vi "GetType.vi"(8 "error in (no error)":errorcluster, 11 "Set Output Voltages Msg":refnum<class "Set Output Voltages Msg.lvclass">) -> (0 "error out":errorcluster, 2 "Data Sample":variant, 3 "Set Output Voltages Msg":refnum<class "Set Output Voltages Msg.lvclass">)   [LabVIEW 2015, in "BNT_DAQmx.lvlib" / "Set Output Voltages Msg.lvclass"]
uses:
  Set Output Voltages Msg.lvclass
  Set Output Voltages Msg.lvclass/Set Output Voltages Msg.ctl
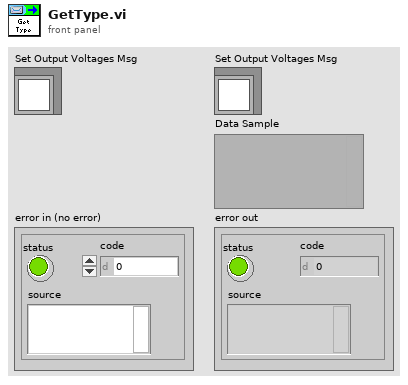
[diagram p1: front panel]
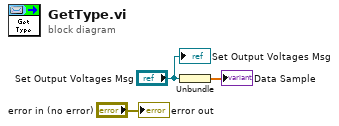
[diagram p0: block diagram]
diagram:
  n1 = Unbundle("Set Output Voltages Msg") -> (→"Data Sample":dbl[unit][])
  "error out" <- "error in (no error)"
  "Set Output Voltages Msg" <- "Set Output Voltages Msg"
